vi "Find XML Node.vi"(8 "error in (no error)":errorcluster, 10 "Node Name":string, 11 "Refnum in":refnum<k20>) -> (0 "error out":errorcluster, 2 "Node":refnum<k20>, 3 "Refnum out":refnum<k20>)   [LabVIEW 2015]
uses:
  <vilib>/xml/Close Reference(Node).vi
  <resource>/objmgr/DOMUserDefRef.rc
  <vilib>/xml/NI_XML.lvlib
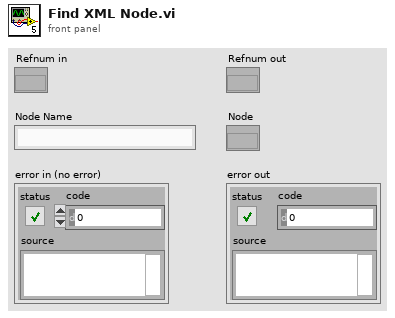
[diagram p1: front panel]
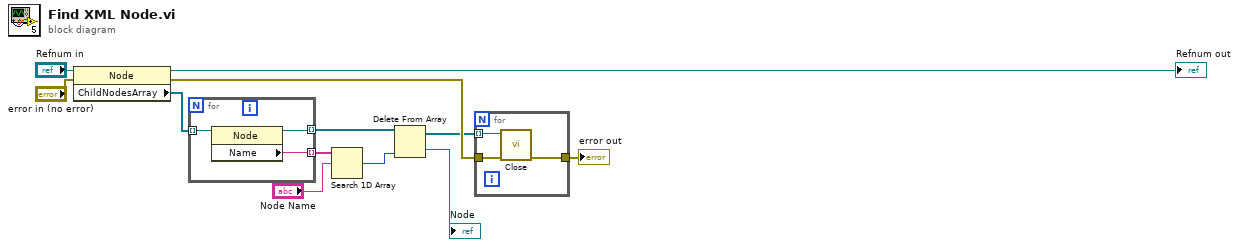
[diagram p0: block diagram]
diagram:
  n1 = property class="Node"(reference="Refnum in", error in="error in (no error)") -> (reference out=→"Refnum out":refnum<k20>, error out=w9:errorcluster, "ChildNodesArray"=w4:refnum<k20>[])
  n2 = for {
    tunnel: w4 -> [w14] mode=indexing
    tunnel: [w15] -> w6 mode=indexing
    tunnel: [w13] -> w11 mode=indexing
    n3 = property class="Node"(reference=w14) -> (reference out=w15:refnum<k20>, "Name"=w13:string)  [unwired: 1 in, 1 out]
  }
  n4 = Search 1D Array(1D array=w11, element="Node Name") -> (index of element=w7:i32)  [unwired: 1 in]
  n5 = Delete From Array(array=w6, index=w7) -> (deleted portion=→"Node":refnum<k20>, array with subset deleted=w8:refnum<k20>[])  [unwired: 1 in]
  n6 = for {
    tunnel: w8 -> [w18] mode=indexing
    tunnel: w9 -> [w17]
    tunnel: [w16] -> w12
    n7 = call-poly <vilib>:"Close.vi"("error in (no error)"=w17, "node"=w18) -> ("error out"=w16:errorcluster)  [unwired: 7 in]
  }
  "error out" <- w12
